vi "Set Dac New 2.vi"(0 "DATA (V)":dbl=5000.0 min=-5000.0 max=5000.0 step=0.001 format="%.2f", 1 "DAC nr":u8=1) -> ()   [LabVIEW 2011]
uses:
  Visa name1.vi
panel:
  out "DATA (hexadecimaal)":u16=65535 format="%.0x"
  out "DATA (decimaal)":u16=65535
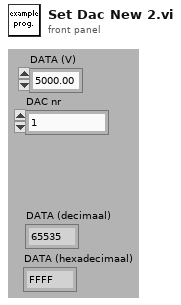
[diagram p1: front panel]
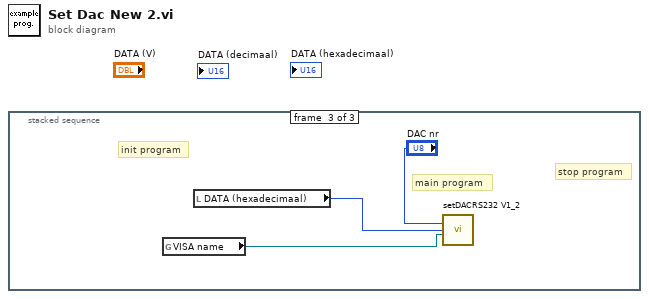
[diagram p0: block diagram]
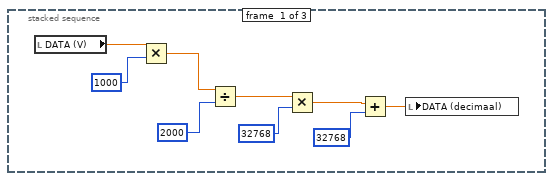
[diagram p2: hidden frame]
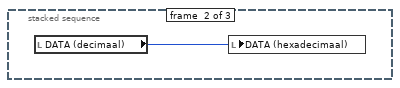
[diagram p3: hidden frame]
diagram:
  n1 = stacked-sequence {
    frame #0 {
      n2 = local read "DATA (V)"() -> (w2:dbl)
      n3 = Multiply(x=w2, y=1000) -> (x*y=w3:dbl)
      n4 = Divide(x=w3, y=2000) -> (x/y=w5:dbl)
      n5 = Multiply(x=w5, y=32768) -> (x*y=w7:dbl)
      n6 = Add(x=w7, y=32768) -> (x+y=w9:dbl)
      n7 = local write "DATA (decimaal)"(w9) -> ()
    }
    frame #1 {
      n8 = local read "DATA (decimaal)"() -> (w10:u16)
      n9 = local write "DATA (hexadecimaal)"(w10) -> ()
    }
    frame #2 {
      # "stop program"
      # "main program"
      # "init program"
      n10 = global read "Visa name1.vi" "VISA name"() -> (w11:refnum<visa-resource-name>)
      n11 = local read "DATA (hexadecimaal)"() -> (w12:u16)
      n12 = call "setDACRS232 V1_2.vi"("VISA resource name IN"=w11, "DATA (hexadecimaal)"=w12, "DAC nr"="DAC nr") -> ()  [unwired: 2 in, 2 out]
    }
  }
